vi "Util_ConvertArrayOfStringPathsToArrayOfPaths.vi"(1 "StringPaths":string[](array[string])) -> (0 "Paths Out":path[](array[path]))   [LabVIEW 2014]
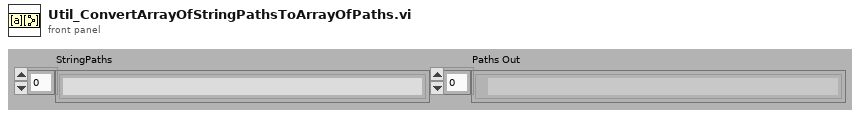
[diagram p1: front panel]
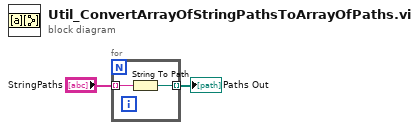
[diagram p0: block diagram]
diagram:
  n1 = for {
    tunnel: "StringPaths" -> [w4] mode=indexing
    tunnel: [w3] -> w1 mode=indexing
    n2 = String To Path(string=w4) -> (path=w3:path)
  }
  "Paths Out" <- w1
